vi "Launch Icon Editor.vi"(8 "error in (no error)":errorcluster, 11 "Icon in":refnum<class "Icon.lvclass">) -> (0 "error out":errorcluster, 3 "Icon out":refnum<class "Icon.lvclass">, 4 "Canceled?":bool)   [LabVIEW 2020, in "LabVIEW Icon API.lvlib"]
doc: "Launches programmatically the Icon Editor. \nThe LabVIEW Icon class data is fully restored in the Icon Editor. When the user clicks on OK, the updated LabVIEW Icon class data is returned.\nIf the user cancels the Icon Editor dialog, the original LabVIEW Icon data is returned."
uses:
  <vilib>/LabVIEW Icon API/LabVIEW Icon API.lvlib
  <vilib>/LabVIEW Icon API/lv_icon/Classes/Icon/Icon.lvclass
  <resource>/plugins/lv_icon.lvlibp
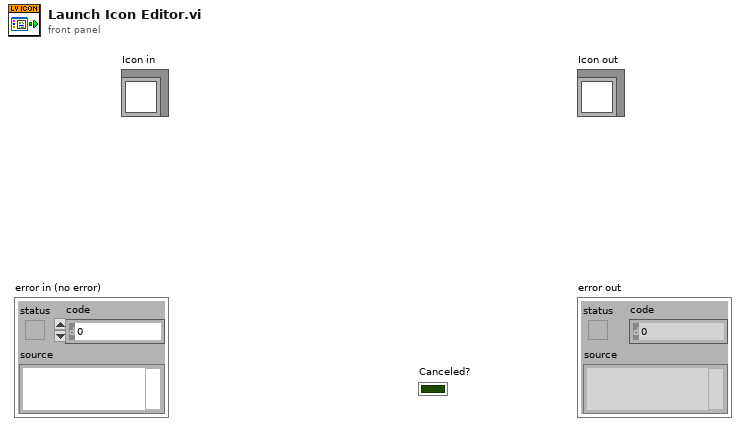
[diagram p1: front panel]
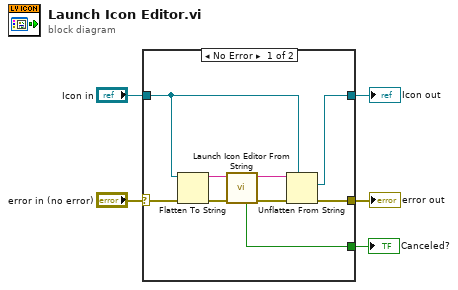
[diagram p0: block diagram]
diagram:
  n1 = case shown="No Error" "error in (no error)" {
    selector: "error in (no error)" -> [w14 w16]
    tunnel: [w6 w16] -> w4
    tunnel: "Icon in" -> [w8 w15]
    tunnel: [w7 w15] -> w2
    tunnel: [w9 _] -> w1
    frame No Error {
      n2 = Flatten To String(anything=w8, error in (no error)=w14) -> (data string=w12:string, error out=w13:errorcluster)  [unwired: 2 in, 1 out]
      n3 = call <resource>:"Launch Icon Editor From String.vi"("error in (no error)"=w13, "Flattened Icon.lvclass in"=w12) -> ("error out"=w11:errorcluster, "Flattened Icon.lvclass out"=w10:string, "Canceled?"=w9:bool)  [unwired: 7 in]
      n4 = Unflatten From String(type=w8, binary string=w10, error in (no error)=w11) -> (value=w7:refnum<class "Icon.lvclass">, error out=w6:errorcluster)  [unwired: 2 in, 1 out]
    }
    frame Error {
    }
  }
  "error out" <- w4
  "Icon out" <- w2
  "Canceled?" <- w1
